vi "CheckVI.vi"(8 "error in (no error)":errorcluster, 11 "VI ref":refnum<vi>) -> (0 "error out":errorcluster, 3 "VI ref out":refnum<vi>)   [LabVIEW 2017, in "MessageGen.lvlib"]
uses:
  <vilib>/addons/InsightCM/MessageBus/CodeGen/MessageGen.lvlib
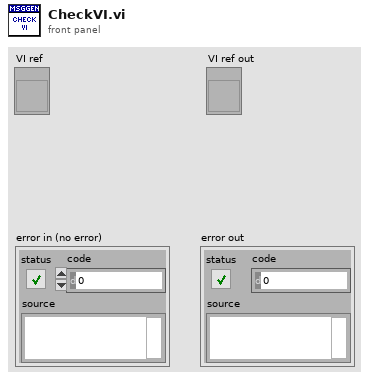
[diagram p1: front panel]
types:
  T1 = enum32{"Bad", "Idle", "Run top level", "Running"}
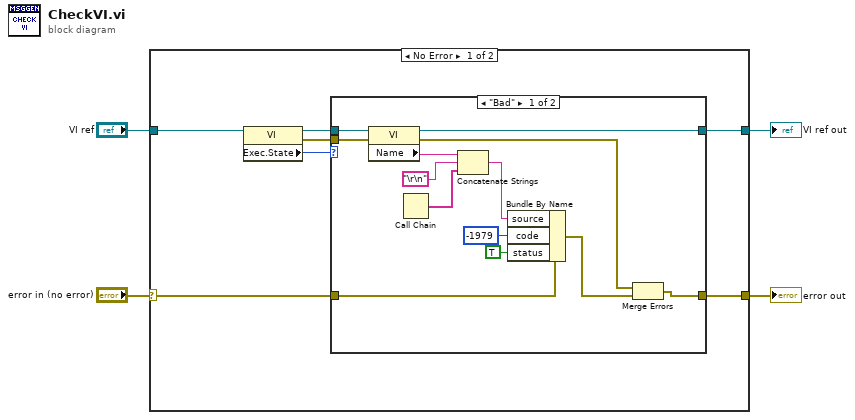
[diagram p0: block diagram]
diagram:
  n1 = case shown="No Error" "error in (no error)" {
    selector: "error in (no error)" -> [w5 w28]
    tunnel: [w11 w28] -> w4
    tunnel: [w10 w27] -> w3
    tunnel: "VI ref" -> [w9 w27]
    frame No Error {
      n2 = property class="VI"(reference=w9) -> (reference out=w8:refnum<vi>, error out=w6:errorcluster, "Exec.State"=w7:T1)  [unwired: 1 in]
      n3 = case shown="\"Bad\"" w7 {
        tunnel: [w12 w25] -> w11
        tunnel: w5 -> [w23 w25]
        tunnel: [w20 w26] -> w10
        tunnel: w8 -> [w24 w26]
        tunnel: w6 -> [w15 _]
        frame "Bad" {
          n4 = property class="VI"(reference=w24, error in=w15) -> (reference out=w20:refnum<vi>, error out=w14:errorcluster, "Name"=w19:string)
          n5 = Call Chain() -> (call chain=w17:string[])
          n6 = Concatenate Strings(w19, "\r\n", w17) -> (w18:string)
          n7 = Bundle By Name(cluster=w23, "source"=w18, "code"=-1979, "status"=TRUE) -> (w13:errorcluster)
          n8 = Merge Errors(w14, w13) -> (w12:errorcluster)
        }
        frame "Idle", Default {
        }
      }
    }
    frame Error {
    }
  }
  "error out" <- w4
  "VI ref out" <- w3
